vi "serial-read-subVi.vi"(8 "error in":errorcluster, 10 "state":string, 11 "VISA resource name":refnum<visa-resource-name>="COM22") -> (0 "error out":errorcluster, 2 "all-sensor-data":T4 {"CD4"."CD3: CO2 (ppm)" format="%.2f"; "CD3"."CD3: CO2 (ppm)" format="%.2f"; "RHT4"."Humidity (%)" format="%.2f"; "RHT4"."Temp (degC)" format="%.2f"; "RHT5"."Humidity (%)" format="%.2f"; "RHT5"."Temp (degC)" format="%.2f"; "CD2"."Humidity (%)" format="%.2f"; "CD2"."Temp (degC)" format="%.2f"; "CD2"."CO2 (ppm)" format="%.2f"; "RHT3"."Humidity (%)" format="%.2f"; "RHT3"."Temp (degC)" format="%.2f"; "CD6"."CD3: CO2 (ppm)" format="%.2f"; "RHT6"."Humidity (%)" format="%.2f"; "RHT6"."Temp (degC)" format="%.2f"; "CD5"."CD3: CO2 (ppm)" format="%.2f"; "CD1"."Humidity (%)" format="%.2f"; "CD1"."Temp (degC)" format="%.2f"; "CD1"."CO2 (ppm)" format="%.2f"}, 3 "VISA resource out":refnum<visa-resource-name>)   [LabVIEW 2021]
uses:
  all-sensor-data.ctl
  SCD41.ctl
  STC31.ctl
  SHT41.ctl
  <vilib>/Instr/_visa.llb/VISA Configure Serial Port (Instr).vi
panel:
  out "RHT4":T1 {"Humidity (%)" format="%.2f"; "Temp (degC)" format="%.2f"}
  out "RHT3":T1 {"Humidity (%)" format="%.2f"; "Temp (degC)" format="%.2f"}
  out "RHT6":T1 {"Humidity (%)" format="%.2f"; "Temp (degC)" format="%.2f"}
  out "RHT5":T1 {"Humidity (%)" format="%.2f"; "Temp (degC)" format="%.2f"}
  out "CD6":T2 {"CD3: CO2 (ppm)" format="%.2f"}
  out "CD5":T2 {"CD3: CO2 (ppm)" format="%.2f"}
  out "CD4":T2 {"CD3: CO2 (ppm)" format="%.2f"}
  out "CD3":T2 {"CD3: CO2 (ppm)" format="%.2f"}
  out "CD2":T3 {"Humidity (%)" format="%.2f"; "Temp (degC)" format="%.2f"; "CO2 (ppm)" format="%.2f"}
  out "CD1":T3 {"Humidity (%)" format="%.2f"; "Temp (degC)" format="%.2f"; "CO2 (ppm)" format="%.2f"}
  out "Num Samples":i32
  out "data string array":string[](array[string])
  out "read buffer":string
  out "Bytes Returned":u32
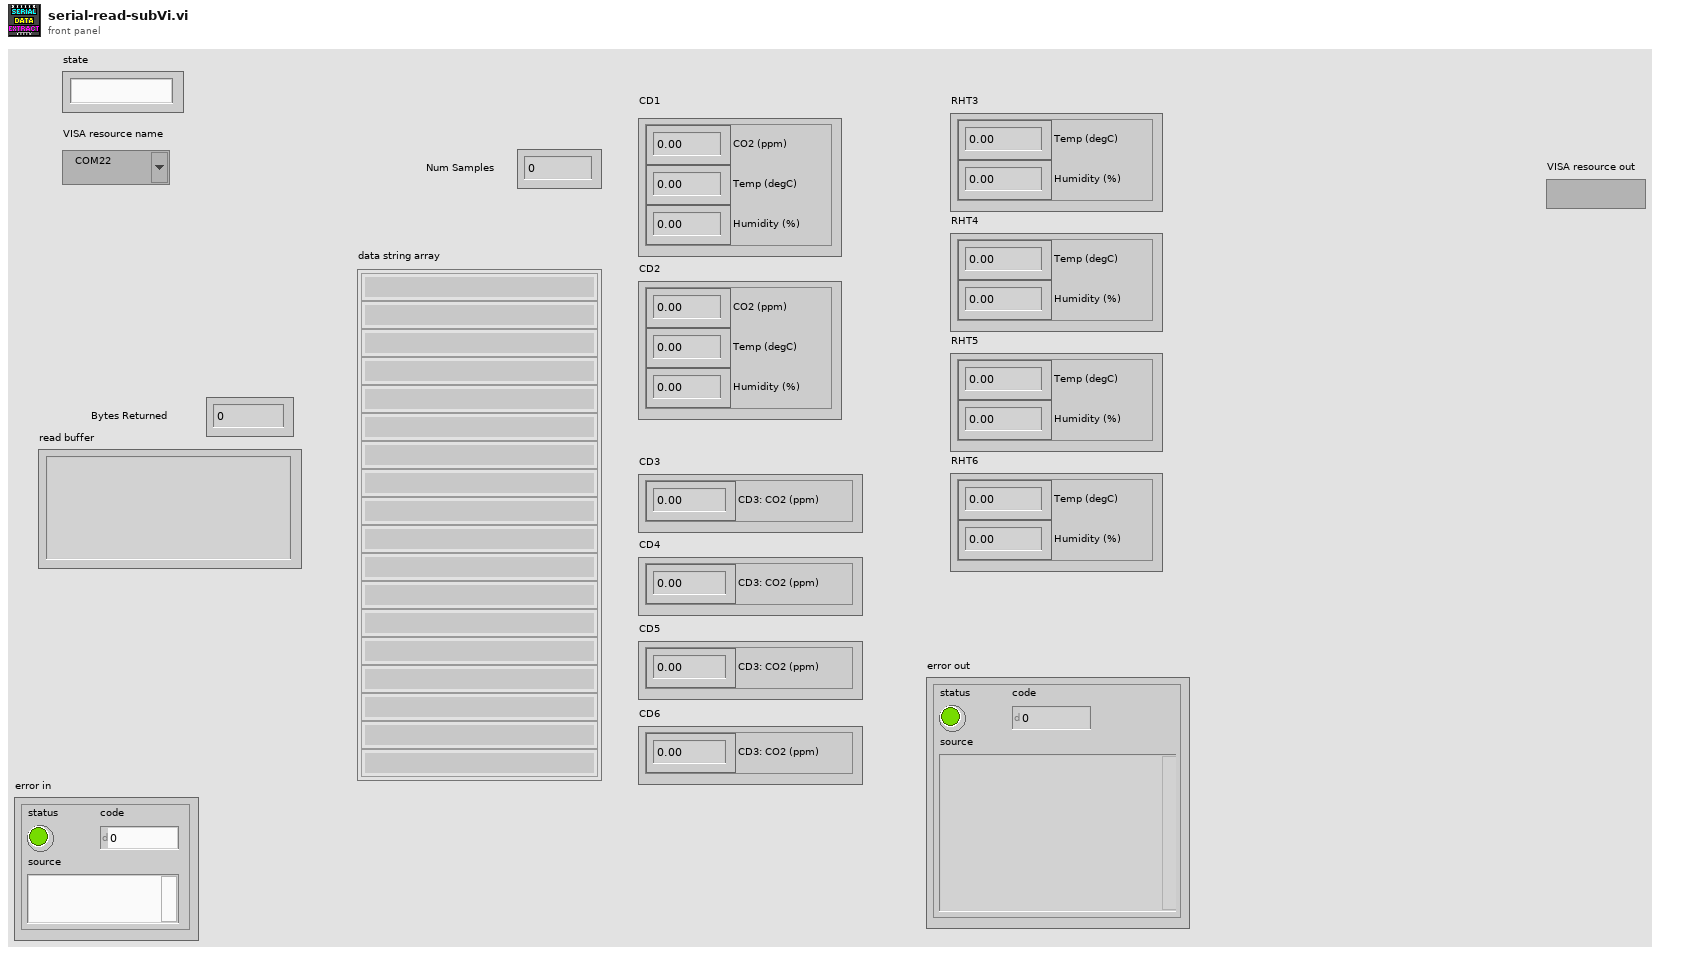
[diagram p1: front panel]
types:
  T1 = typedef "SHT41.ctl" = cluster{"Temp (degC)":dbl, "Humidity (%)":dbl}
  T2 = typedef "STC31.ctl" = cluster{"CD3: CO2 (ppm)":dbl}
  T3 = typedef "SCD41.ctl" = cluster{"CO2 (ppm)":dbl, "Temp (degC)":dbl, "Humidity (%)":dbl}
  T4 = typedef "all-sensor-data.ctl" = cluster{"CD1":T3, "CD2":T3, "CD3":T2, "CD4":T2, "CD5":T2, "CD6":T2, "RHT3":T1, "RHT4":T1, "RHT5":T1, "RHT6":T1}
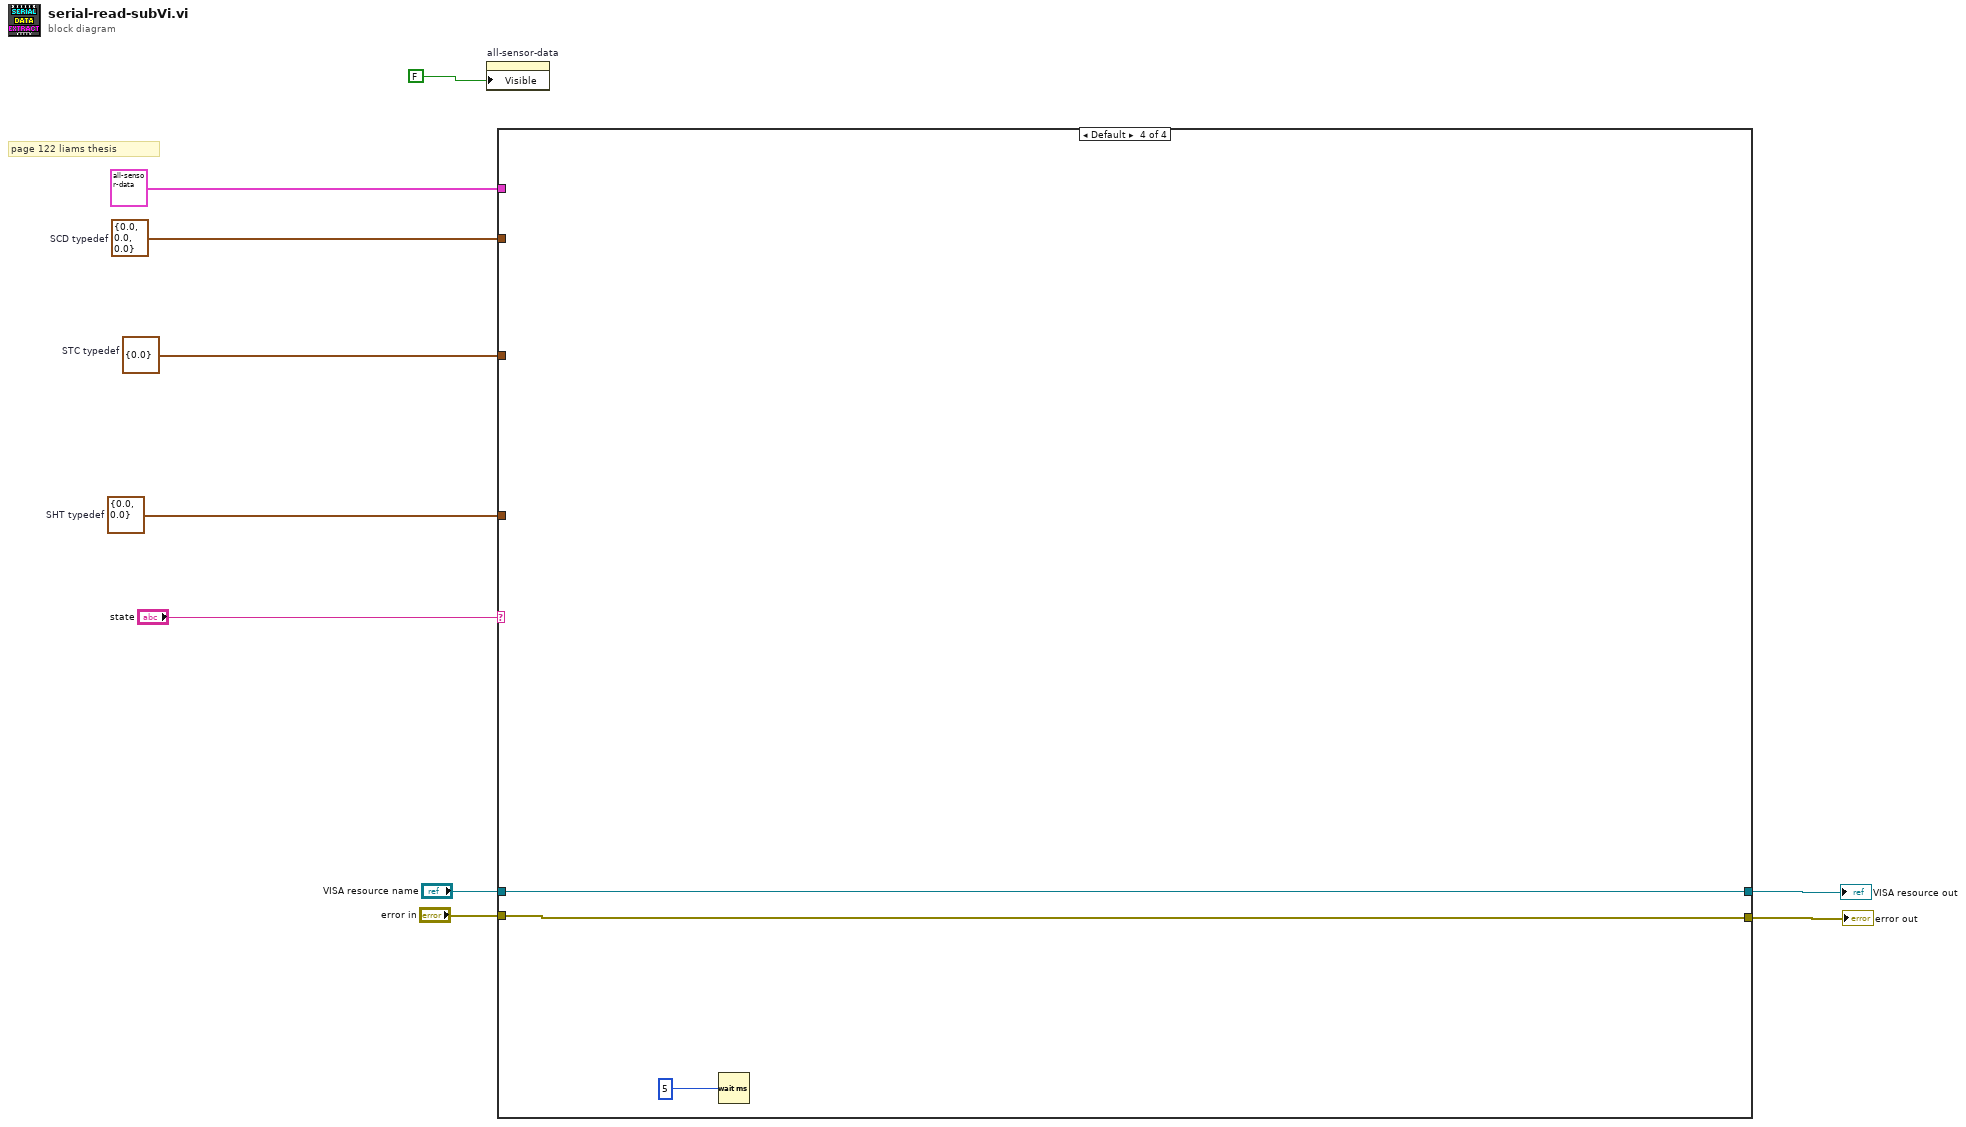
[diagram p0: block diagram]
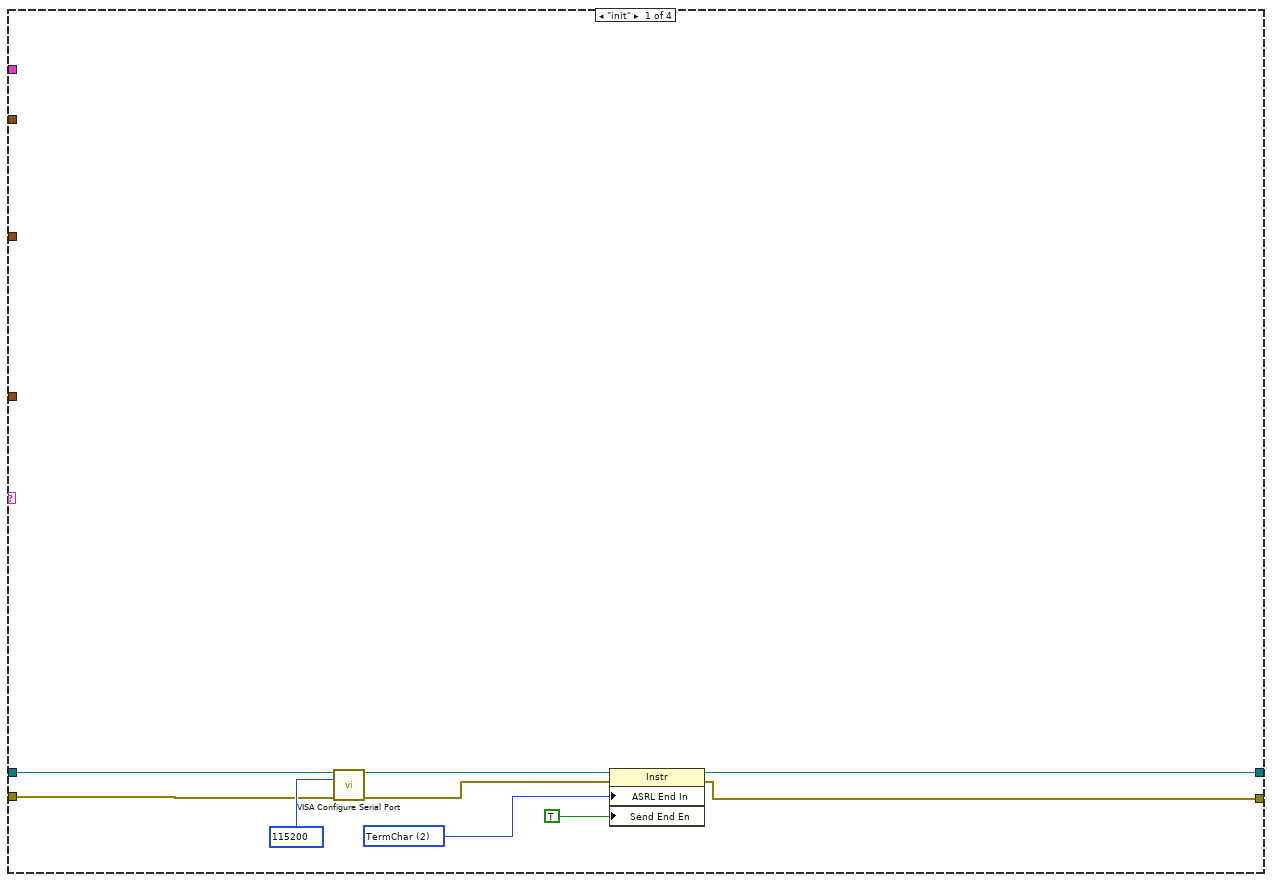
[diagram p2: hidden frame]
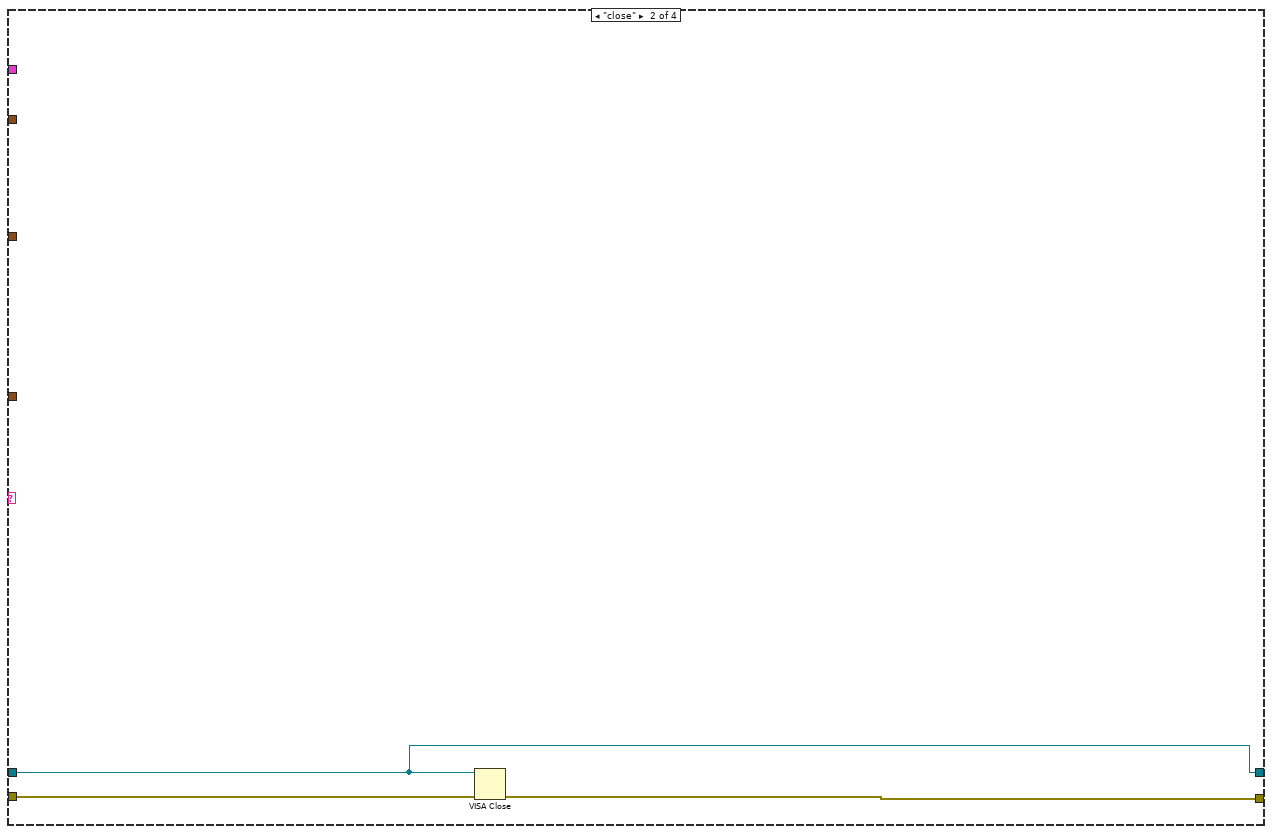
[diagram p3: hidden frame]
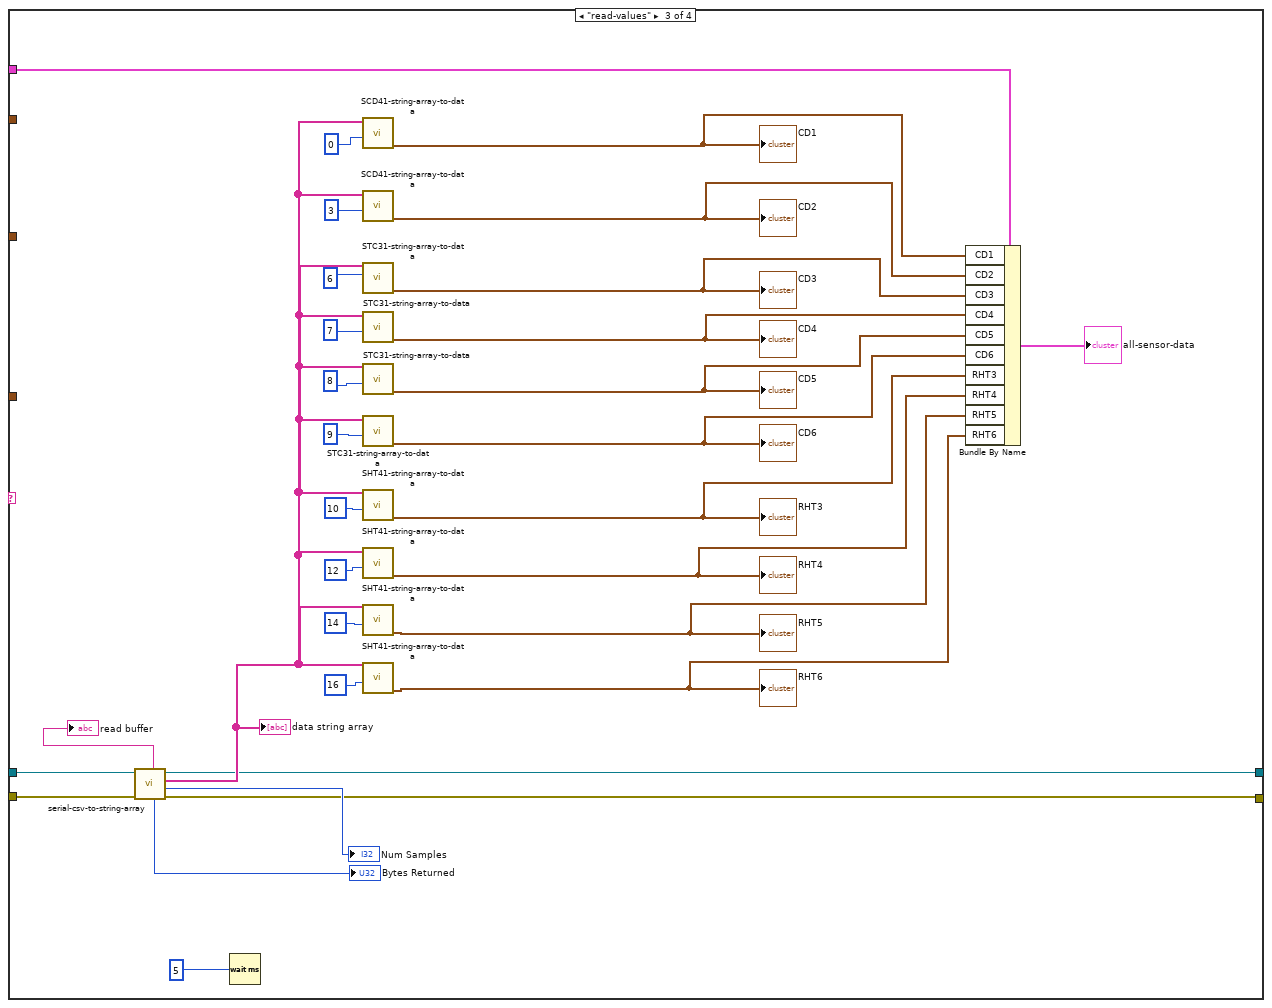
[diagram p4: hidden frame]
diagram:
  w6 = T1 {"Temp (degC)"=0.0, "Humidity (%)"=0.0}  # SHT typedef
  w7 = T2 {"CD3: CO2 (ppm)"=0.0}  # STC typedef
  w8 = T3 {"CO2 (ppm)"=0.0, "Temp (degC)"=0.0, "Humidity (%)"=0.0}  # SCD typedef
  # "page 122 liams thesis"
  n1 = property on="all-sensor-data" class="Clust (strict)"("Visible"=FALSE) -> ()  [unwired: 2 in, 2 out]
  n2 = case shown="Default" "state" {
    tunnel: "VISA resource name" -> [w14 w20 w40 w55]
    tunnel: w8 -> [_ _ _ _]
    tunnel: w7 -> [_ _ _ _]
    tunnel: w6 -> [_ _ _ _]
    tunnel: T4 {"CD1"={"CO2 (ppm)"=0.0, "Temp (degC)"=0.0, "Humidity (%)"=0.0}, "CD2"={"CO2 (ppm)"=0.0, "Temp (degC)"=0.0, "Humidity (%)"=0.0}, "CD3"={"CD3: CO2 (ppm)"=0.0}, "CD4"={"CD3: CO2 (ppm)"=0.0}, "CD5"={"CD3: CO2 (ppm)"=0.0}, "CD6"={"CD3: CO2 (ppm)"=0.0}, "RHT3"={"Temp (degC)"=0.0, "Humidity (%)"=0.0}, "RHT4"={"Temp (degC)"=0.0, "Humidity (%)"=0.0}, "RHT5"={"Temp (degC)"=0.0, "Humidity (%)"=0.0}, "RHT6"={"Temp (degC)"=0.0, "Humidity (%)"=0.0}} ("all-data") -> [_ _ w42 _]
    tunnel: "error in" -> [w13 w22 w39 w54]
    tunnel: [w12 w21 w23 w54] -> w3
    tunnel: [w11 w20 w24 w55] -> w2
    frame "init" {
      w17 = u16 2 items=["None", "Last Bit", "TermChar"] ("Serial Settings:End Mode for Reads")
      n3 = call-poly "VISA Configure Serial Port"("VISA resource name"=w14, "baud rate (9600)"=u32 115200, "error in (no error)"=w13) -> ("VISA resource name out"=w18:refnum<visa-resource-name>, "error out"=w19:errorcluster)  [unwired: 11 in]
      n4 = property class="Instr"(reference=w18, error in=w19, "ASRL End In"=w17, "Send End En"=TRUE ("Message Based Settings:Send End Enable")) -> (reference out=w11:refnum<visa-resource-name>, error out=w12:errorcluster)
    }
    frame "close" {
      n5 = VISA Close(VISA resource name=w20, error in (no error)=w22) -> (error out=w21:errorcluster)
    }
    frame "read-values" {
      n6 = call "serial-csv-to-string-array.vi"("error in (no error)"=w39, "VISA Refnum in"=w40) -> ("error out"=w23:errorcluster, "Num Samples Reported"=→"Num Samples":i32, "data string array"=w38:string[], "VISA Refnum out"=w24:refnum<visa-resource-name>, "Bytes Returned"=→"Bytes Returned":u32, "read buffer"=→"read buffer":string)  [unwired: 4 in]
      "data string array" <- w38
      n7 = Wait (ms)(milliseconds to wait=u32 5) -> ()  [unwired: 1 out]
      n8 = call "SCD41-string-array-to-data.vi"("Starting Index"=0, "Data In (string array)"=w38) -> ("SCD41: data output"=w37:T3)  [unwired: 6 in, 3 out]
      "CD1" <- w37
      n9 = call "SCD41-string-array-to-data.vi"("Starting Index"=3, "Data In (string array)"=w38) -> ("SCD41: data output"=w36:T3)  [unwired: 6 in, 3 out]
      "CD2" <- w36
      n10 = call "STC31-string-array-to-data.vi"("Starting Index"=6 ("index"), "Data In (string array)"=w38) -> ("STC31: data output"=w35:T2)  [unwired: 7 in, 2 out]
      "CD3" <- w35
      n11 = call "STC31-string-array-to-data.vi"("Starting Index"=7, "Data In (string array)"=w38) -> ("STC31: data output"=w34:T2)  [unwired: 7 in, 2 out]
      "CD4" <- w34
      n12 = call "STC31-string-array-to-data.vi"("Starting Index"=8, "Data In (string array)"=w38) -> ("STC31: data output"=w33:T2)  [unwired: 7 in, 2 out]
      "CD5" <- w33
      n13 = call "STC31-string-array-to-data.vi"("Starting Index"=9, "Data In (string array)"=w38) -> ("STC31: data output"=w32:T2)  [unwired: 7 in, 2 out]
      "CD6" <- w32
      n14 = call "SHT41-string-array-to-data.vi"("Starting Index"=10, "Data In (string array)"=w38) -> ("SHT41: data output"=w31:T1)  [unwired: 7 in, 2 out]
      "RHT3" <- w31
      n15 = call "SHT41-string-array-to-data.vi"("Starting Index"=12, "Data In (string array)"=w38) -> ("SHT41: data output"=w30:T1)  [unwired: 7 in, 2 out]
      "RHT4" <- w30
      n16 = call "SHT41-string-array-to-data.vi"("Starting Index"=14, "Data In (string array)"=w38) -> ("SHT41: data output"=w29:T1)  [unwired: 7 in, 2 out]
      "RHT5" <- w29
      n17 = call "SHT41-string-array-to-data.vi"("Starting Index"=16, "Data In (string array)"=w38) -> ("SHT41: data output"=w28:T1)  [unwired: 7 in, 2 out]
      "RHT6" <- w28
      n18 = Bundle By Name(cluster=w42, "CD1"=w37, "CD2"=w36, "CD3"=w35, "CD4"=w34, "CD5"=w33, "CD6"=w32, "RHT3"=w31, "RHT4"=w30, "RHT5"=w29, "RHT6"=w28) -> (→"all-sensor-data":T4)
    }
    frame Default {
      n19 = Wait (ms)(milliseconds to wait=u32 5) -> ()  [unwired: 1 out]
    }
  }
  "error out" <- w3
  "VISA resource out" <- w2
